vi "PeakCheck.vi"(8 "REF계산값":dbl, 9 "거리 배열":dbl[](array[numeric]), 10 "LOG(AS)-LOG(S)":dbl[](array[numeric]), 11 "LOG(AS-S)":dbl[](array[numeric])) -> (7 "T.H 값":dbl)   [LabVIEW 2020]
panel:
  in  "T.H 가중치":sgl(slide)=0.01 min=0.001 max=0.01 step=0.001 scale=0.0..0.01
  in  "테스트 Gain":dbl=1.0
  out "XY Graph":cluster{"Y":dbl[], "Y":dbl[]}[](graph) caption="XY 그래프"
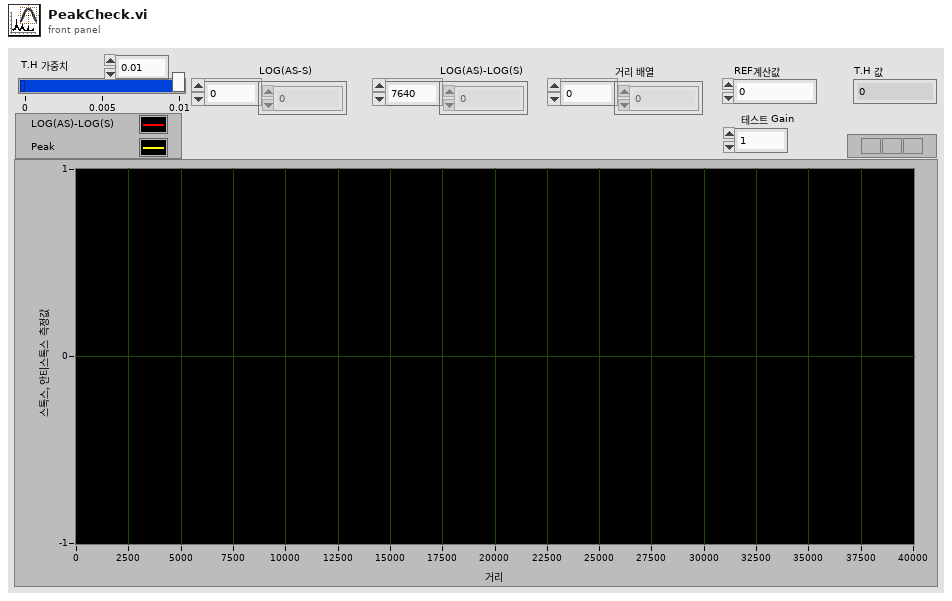
[diagram p1: front panel]
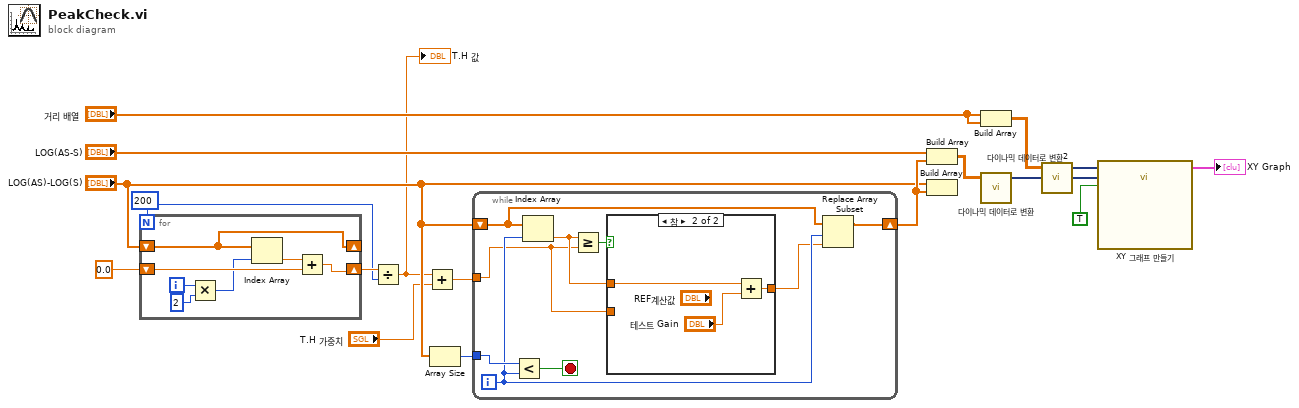
[diagram p0: block diagram]
diagram:
  w7 = 200
  n1 = for {
    N: w7 -> [_]
    shift-right: [w22] -> w9
    shift-left: 0.0 -> [w23]
    shift-right: [w21] -> _
    shift-left: "LOG(AS)-LOG(S)" -> [w21]
    i -> [w20]
    n2 = Multiply(x=w20, y=2) -> (x*y=w18:i32)
    n3 = Index Array(array=w21, index=w18) -> (element=w24:dbl)
    n4 = Add(x=w24, y=w23) -> (x+y=w22:dbl)
  }
  n5 = Divide(x=w9, y=w7) -> (x/y=w3:dbl)
  "T.H 값" <- w3
  n6 = Add(x=w3, y="T.H 가중치") -> (x+y=w4:dbl)
  n7 = Array Size(array="LOG(AS)-LOG(S)") -> (size(s)=w8:i32)
  n8 = while {
    tunnel: w8 -> [w33]
    shift-right: [w26] -> w12
    shift-left: "LOG(AS)-LOG(S)" -> [w29]
    tunnel: w4 -> [w25]
    i -> [w28]
    stop <- w32 stop-if-true
    n9 = Less?(x=w33, y=w28) -> (x < y?=w32:bool)
    n10 = Index Array(array=w29, index=w28) -> (element=w30:dbl)
    n11 = Greater Or Equal?(x=w30, y=w25) -> (x >= y?=w31:bool)
    n12 = case shown="참" w31 {
      tunnel: w30 -> [w34 w37]
      tunnel: [w34 w36] -> w27
      tunnel: w25 -> [_ _]
      frame False {
      }
      frame True {
        n13 = Add(x=w37, y="테스트 Gain") -> (x+y=w36:dbl)
      }
    }
    n14 = Replace Array Subset(array=w29, new element=w27, index=w28) -> (w26:dbl[])
  }
  n15 = Build Array("LOG(AS-S)", w12) -> (w1:dbl[][])
  n16 = Build Array("LOG(AS)-LOG(S)", w12) -> ()  [unwired: 1 out]
  n17 = Build Array("거리 배열", "거리 배열") -> (w13:dbl[][])
  n18 = call "다이나믹 데이터로 변환"("2D Array"=w1) -> ("Dynamic Data Type"=w15:dynamicdata)  [unwired: 3 in]
  n19 = call "다이나믹 데이터로 변환2"("2D Array"=w13) -> ("Dynamic Data Type"=w16:dynamicdata)  [unwired: 3 in]
  n20 = call "XY 그래프 만들기"("Reset"=TRUE, "Y Input"=w15, "X Input"=w16) -> ("XY Graph"=→"XY Graph":cluster{"X":dbl[], "Y":dbl[]}[])  [unwired: 7 in, 1 out]
